vi "Unbundle.vi"(8 "error in (no error)":errorcluster, 11 "Request Data in":refnum<class "Request Data.lvclass">) -> (0 "error out":errorcluster, 1 "Request ID":u32, 2 "Data":refnum<class "Data.lvclass">, 3 "Request Data out":refnum<class "Request Data.lvclass">)   [LabVIEW 2020, in "Publisher.lvlib" / "Request Data.lvclass"]
doc: "Read the Data and Request ID from the Request Data."
uses:
  Request Data.lvclass
  PPL/HDH.Data.Generic.lvlibp/Data.lvclass
  Request Data.lvclass/Request Data.ctl
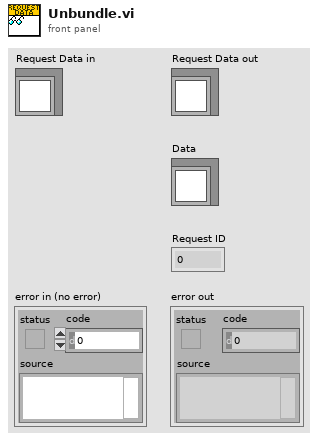
[diagram p1: front panel]
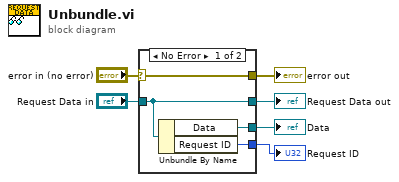
[diagram p0: block diagram]
diagram:
  n1 = case shown="No Error" "error in (no error)" {
    selector: "error in (no error)" -> [w10 w11]
    tunnel: [w10 w11] -> w5
    tunnel: [w9 w12] -> w3
    tunnel: "Request Data in" -> [w9 w12]
    tunnel: [w8 _] -> w2
    tunnel: [w7 _] -> w1
    frame No Error {
      n2 = Unbundle By Name(w9) -> ("Data"=w8:refnum<class "Data.lvclass">, "Request ID"=w7:u32)
    }
    frame Error {
    }
  }
  "error out" <- w5
  "Request Data out" <- w3
  "Data" <- w2
  "Request ID" <- w1
